vi "Insertable array.vi"() -> ()   [LabVIEW 2015]
panel:
  out "Column":i32
  out "Array":dbl[][](array[numeric])
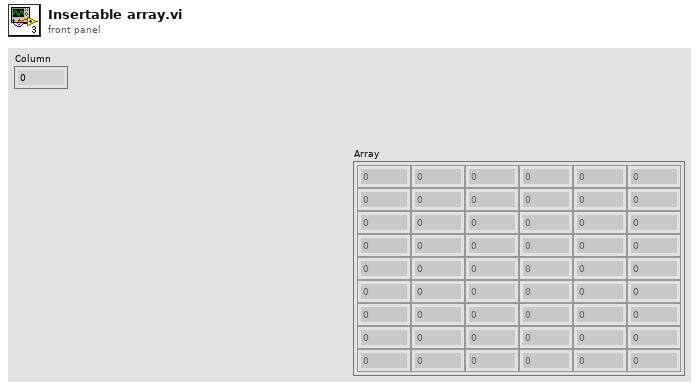
[diagram p1: front panel]
types:
  T1 = typedef "LVPoint32TypeDef.ctl" = cluster{"Horizontal":i32, "Vertical":i32}
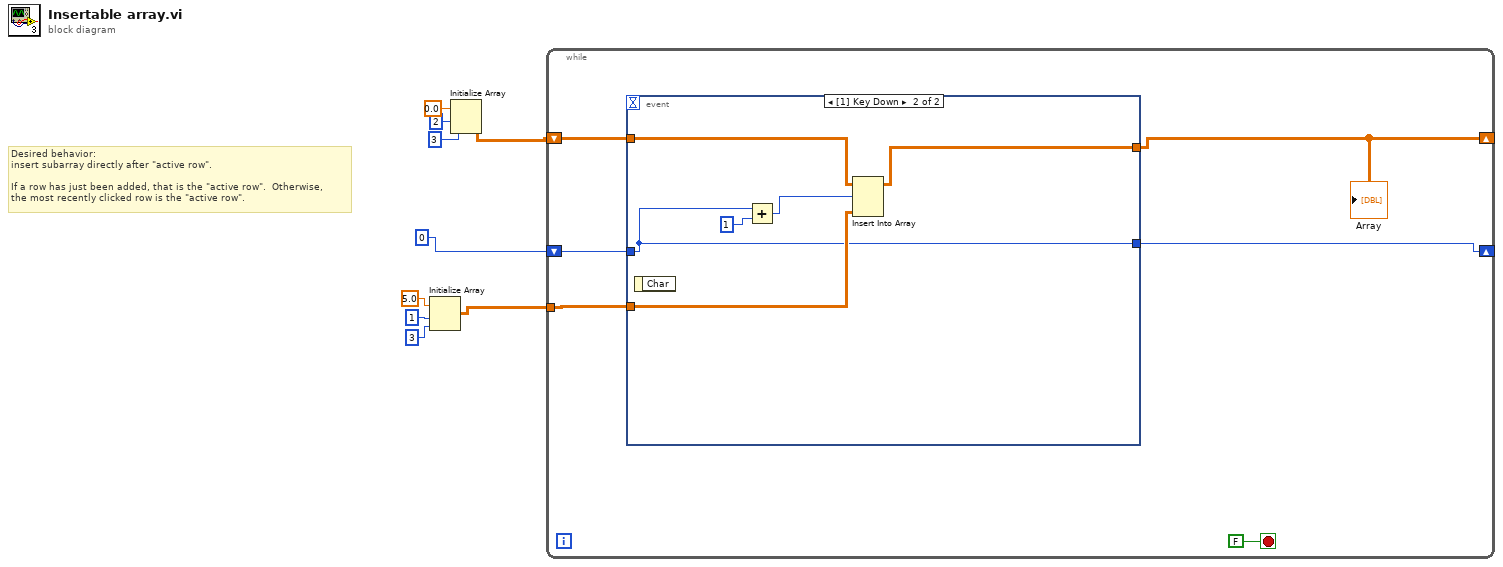
[diagram p0: block diagram]
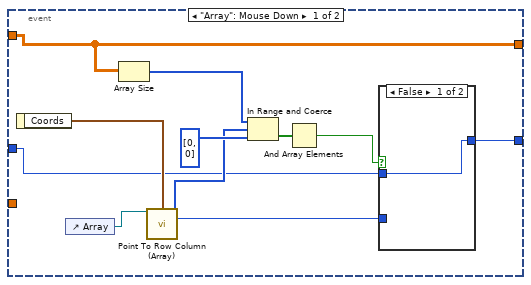
[diagram p2: hidden frame]
diagram:
  # "Desired behavior:\ninsert subarray directly after \"active row\".\n\nIf a row has just been added, that is the \"active row\".  Otherwise,\nthe most recently clicked row is the \"active row\"."
  n1 = Initialize Array(5.0 ("element"), 1 ("dimension size"), 3 ("dimension size")) -> (w2:dbl[][])
  n2 = Initialize Array(0.0 ("element"), 2 ("dimension size"), 3 ("dimension size")) -> (w6:dbl[][])
  n3 = while {
    shift-right: [w14] -> _
    shift-left: w6 -> [w15]
    tunnel: w2 -> [w12]
    shift-right: [w10] -> _
    shift-left: 0 ("dimension size") -> [w11]
    stop <- FALSE stop-if-true
    n4 = event shown="[1] Key Down" {
      selector: _ -> [_ _]
      dyn-events: _ -> [_ _]
      timeout: _ -> [_ _]
      tunnel: [w21 w33] -> w14
      tunnel: w15 -> [w21 w34]
      tunnel: w12 -> [_ w32]
      tunnel: w11 -> [w16 w29]
      tunnel: [w18 w29] -> w10
      event "Array": Mouse Down {
        n5 = event-data() -> ("Coords"=w26:T1)  [unwired: 1 in]
        n6 = control-ref of="Array"() -> (w22:refnum<vi>)
        n7 = Array Size(array=w21) -> (size(s)=w20:i32[])
        n8 = call "Point To Row Column (Array).vi"("reference"=w22, "Coords of Click"=w26) -> ("Clicked Index"=w23:i32[], "Clicked Row"=w17:i32)  [unwired: 8 in, 4 out]
        n9 = In Range and Coerce(upper limit=w20, x=w23, lower limit=i32[] [0, 0]) -> (In Range?=w24:bool[])  [unwired: 1 out]
        n10 = And Array Elements(Boolean array=w24) -> (logical AND=w19:bool)
        n11 = case shown="False" w19 {
          tunnel: [w27 w28] -> w18
          tunnel: w17 -> [_ w28]
          tunnel: w16 -> [w27 _]
          frame False {
          }
          frame True {
          }
        }
      }
      event Key Down {
        n12 = event-data() -> ()  [unwired: 1 in, 1 out]
        n13 = Add(x=w29, y=1) -> (x+y=w30:i32)
        n14 = Insert Into Array(array=w34, index (row)=w30, new element=w32) -> (w33:dbl[][])  [unwired: 1 in]
      }
    }
    "Array" <- w14
  }
